vi "Write States.vi"(8 "error in (no error)":errorcluster, 10 "States":enum16{"Exit", "Halt", "GoTo"}(ring), 11 "ReceivePassInFuturePointTactic in":refnum<class "ReceivePassInFuturePointTactic.lvclass">) -> (0 "error out":errorcluster, 3 "ReceivePassInFuturePointTactic out":refnum<class "ReceivePassInFuturePointTactic.lvclass">)   [LabVIEW 2023, in "ReceivePassInFuturePointTactic.lvclass"]
uses:
  ReceivePassInFuturePointTactic.lvclass
  ReceivePassInFuturePointTactic.lvclass/ReceivePassInFuturePointTactic.ctl
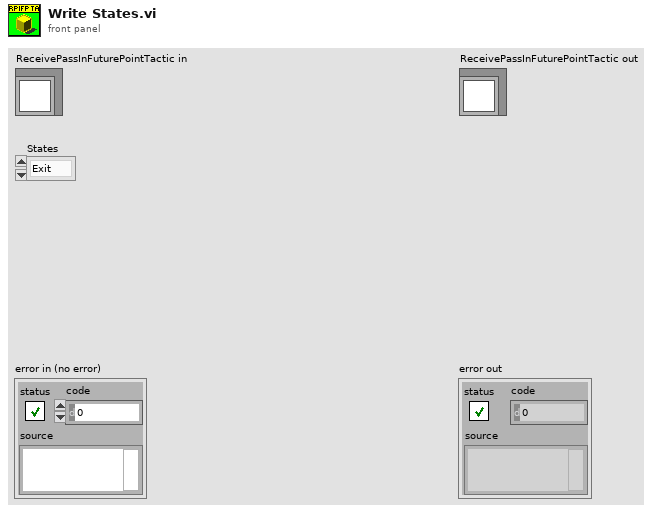
[diagram p1: front panel]
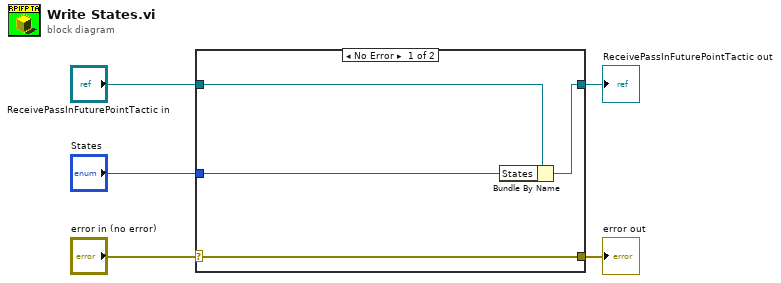
[diagram p0: block diagram]
diagram:
  n1 = case shown="No Error" "error in (no error)" {
    selector: "error in (no error)" -> [w9 w10]
    tunnel: [w9 w10] -> w4
    tunnel: [w7 w11] -> w2
    tunnel: "ReceivePassInFuturePointTactic in" -> [w8 w11]
    tunnel: "States" -> [w6 _]
    frame No Error {
      n2 = Bundle By Name(cluster=w8, "States"=w6) -> (w7:refnum<class "ReceivePassInFuturePointTactic.lvclass">)
    }
    frame Error {
    }
  }
  "error out" <- w4
  "ReceivePassInFuturePointTactic out" <- w2
